vi "Set configuration chain.vi"(8 "error in (no error)":errorcluster, 9 "class names":string[](array[string]), 10 "configuration":variant[](array[variant]), 11 "Autofocus in":refnum<class "Autofocus.lvclass">) -> (0 "error out":errorcluster, 3 "Autofocus out":refnum<class "Autofocus.lvclass">)   [LabVIEW 2012, in "Autofocus.lvclass"]
uses:
  Autofocus.lvclass
  <vilib>/Distrio/Murmex/Murmex/Murmex.lvclass
  Autofocus.lvclass/Autofocus.ctl
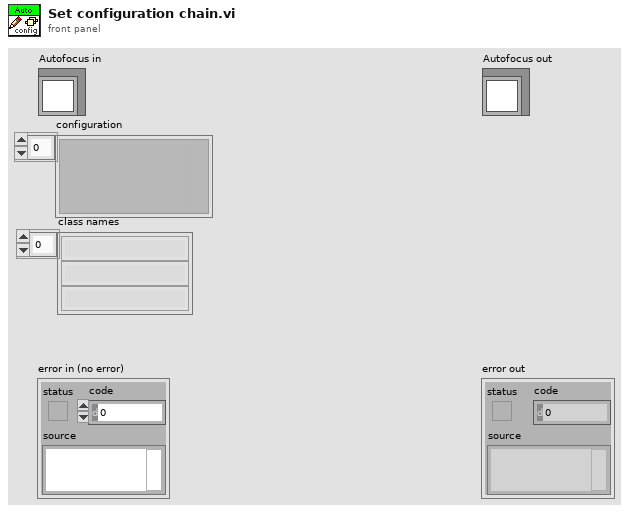
[diagram p1: front panel]
types:
  T1 = typedef "Autofocus.lvclass/configuration cluster.ctl" = cluster{"Camera component name":string, "Tomo component name":string, "Epsilon (HC)":dbl, "Epsilon (GS)":dbl, "Number of subregions":T2, "Sample stage component name":string, "Image File Path":path, "Reporting folder":path, "Default stage speed":dbl[unit]}
  T2 = typedef "Autofocus.lvclass/number of subregions.ctl" = i32
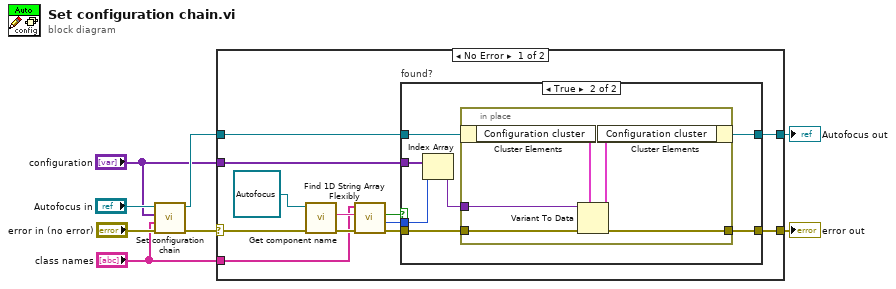
[diagram p0: block diagram]
diagram:
  n1 = call-parent "Set configuration chain.vi"("error in (no error)"="error in (no error)", "class names"="class names", "configuration"="configuration", "Murmex in"="Autofocus in") -> ("error out"=w6:errorcluster, "Murmex out"=w5:refnum<class "Autofocus.lvclass">)  [unwired: 6 in]
  n2 = case shown="No Error" w6 {
    selector: w6 -> [w18 w35]
    tunnel: w5 -> [w11 w36]
    tunnel: "configuration" -> [w12 _]
    tunnel: "class names" -> [w16 _]
    tunnel: [w10 w36] -> w2
    tunnel: [w9 w35] -> w1
    frame No Error {
      n3 = call <vilib>:"Get component name.vi"("error in (no error)"=w18, "Murmex in"=refnum<class "Autofocus.lvclass"> refnum ("Autofocus.lvclass")) -> ("error out"=w19:errorcluster, "component name"=w20:string)  [unwired: 7 in, 1 out]
      n4 = call <vilib>:"Find 1D String Array Flexibly.vi"("error in (no error)"=w19, "element"=w20, "array"=w16) -> ("error out"=w15:errorcluster, "index of element"=w13:i32, "found?"=w14:bool)  [unwired: 6 in]
      n5 = case "found?" shown="True" w14 {
        tunnel: w13 -> [_ w27]
        tunnel: w15 -> [w22 w26]
        tunnel: [w22 w25] -> w9
        tunnel: [w21 w23] -> w10
        tunnel: w11 -> [w21 w29]
        tunnel: w12 -> [_ w28]
        frame False {
        }
        frame True {
          n6 = Index Array(array=w28, index=w27) -> (element=w24:variant)
          n7 = in-place {
            in-place-border: w26 -> [w34]
            in-place-border: [w33] -> w25
            in-place-border: w24 -> [w30]
            n8 = in-place-cluster #1(w29) -> ("Configuration cluster"=w32:T1)
            n9 = Variant To Data(error in=w34, type=w32, Variant=w30) -> (data=w31:T1, error out=w33:errorcluster)
            n10 = in-place-cluster #1("Configuration cluster"=w31) -> (w23:refnum<class "Autofocus.lvclass">)
          }
        }
      }
    }
    frame Error {
    }
  }
  "error out" <- w1
  "Autofocus out" <- w2
